vi "Maui.Config.Create.vi"(8 "error in (no error)":errorcluster, 10 "Owning Class":refnum<class>, 11 "Maui.Config in":refnum<class "Maui.Config.lvclass">) -> (0 "error out":errorcluster, 3 "Maui.Config out":refnum<class "Maui.Config.lvclass">)   [LabVIEW 2020, in "Maui.Config.lvclass"]
uses:
  Maui.Config.lvclass
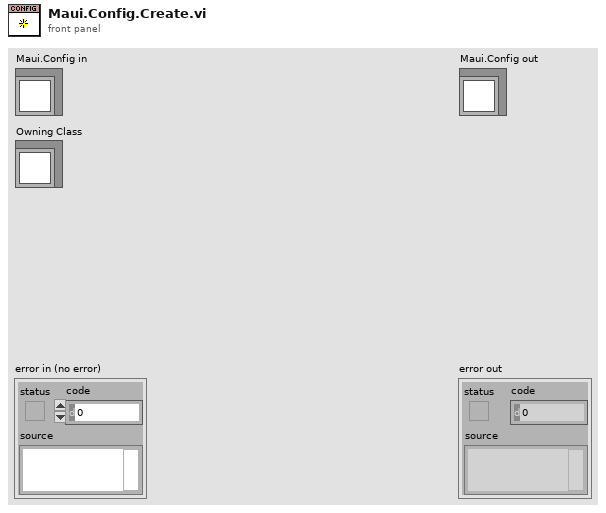
[diagram p1: front panel]
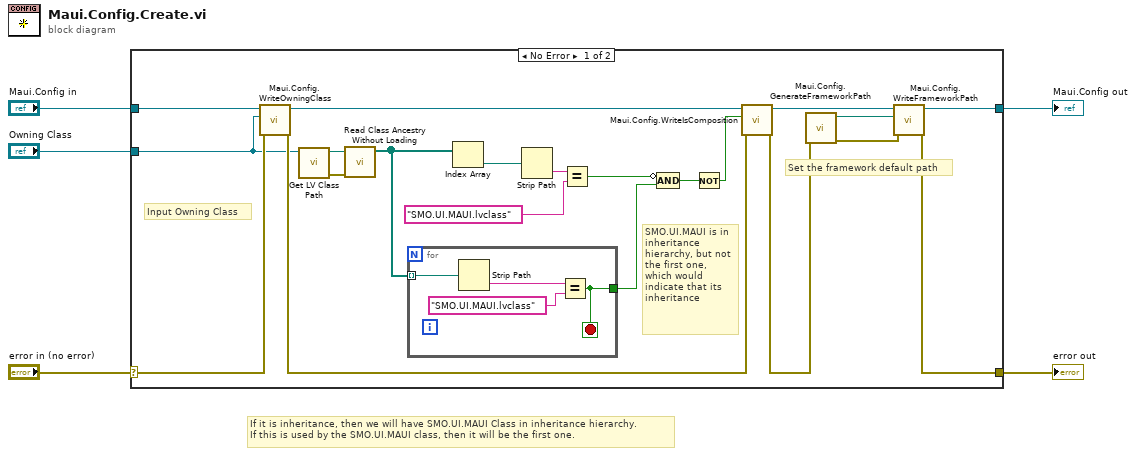
[diagram p0: block diagram]
diagram:
  # "If it is inheritance, then we will have SMO.UI.MAUI Class in inheritance hierarchy.\nIf this is used by the SMO.UI.MAUI class, then it will be the first one."
  n1 = case shown="No Error" "error in (no error)" {
    selector: "error in (no error)" -> [w25 w32]
    tunnel: [w20 w32] -> w4
    tunnel: [w21 w31] -> w2
    tunnel: "Maui.Config in" -> [w26 w31]
    tunnel: "Owning Class" -> [w14 _]
    frame No Error {
      # "SMO.UI.MAUI is in inheritance hierarchy, but not the first one, which would indicate that its inheritance"
      # "Set the framework default path"
      # "Input Owning Class"
      n2 = call "Maui.Config.WriteOwningClass.vi"("error in (no error)"=w25, "Owning Class"=w14, "Maui.Config in"=w26) -> ("error out"=w23:errorcluster, "Maui.Config out"=w24:refnum<class "Maui.Config.lvclass">)  [unwired: 7 in]
      n3 = call <vilib>:"Get LV Class Path.vi"("object"=w14) -> ("error out"=w16:errorcluster, "class path"=w15:path)  [unwired: 9 in]
      n4 = call <vilib>:"Read Class Ancestry Without Loading.vi"("error in (no error)"=w16, "LabVIEW Class Path"=w15) -> ("Class Ancestry"=w13:path[])  [unwired: 8 in, 1 out]
      n5 = for {
        tunnel: [w27] -> w8
        tunnel: w13 -> [w28] mode=indexing
        stop <- w27 stop-if-true
        n6 = Strip Path(path=w28) -> (name=w30:string)  [unwired: 1 out]
        n7 = Equal?(x=w30, y="SMO.UI.MAUI.lvclass") -> (x = y?=w27:bool)
      }
      n8 = Index Array(array=w13) -> (element=w12:path)  [unwired: 1 in]
      n9 = Strip Path(path=w12) -> (name=w11:string)  [unwired: 1 out]
      n10 = Equal?(x=w11, y="SMO.UI.MAUI.lvclass") -> (x = y?=w9:bool)
      n11 = Compound Arithmetic op=AND(invert w9, w8) -> (w7:bool)
      n12 = Not(x=w7) -> (.not. x?=w6:bool)
      n13 = call "Maui.Config.WriteIsComposition.vi"("error in (no error)"=w23, "Composition"=w6, "Maui.Config in"=w24) -> ("error out"=w18:errorcluster, "Maui.Config out"=w22:refnum<class "Maui.Config.lvclass">)  [unwired: 7 in]
      n14 = call "Maui.Config.GenerateFrameworkPath.vi"("error in (no error)"=w18) -> ("error out"=w17:errorcluster, "Framework Path"=w19:path)  [unwired: 8 in, 1 out]
      n15 = call "Maui.Config.WriteFrameworkPath.vi"("error in (no error)"=w17, "Framework Path"=w19, "Maui.Config in"=w22) -> ("error out"=w20:errorcluster, "Maui.Config out"=w21:refnum<class "Maui.Config.lvclass">)  [unwired: 7 in]
    }
    frame Error {
    }
  }
  "error out" <- w4
  "Maui.Config out" <- w2
